vi "Turn Off All Outputs.vi"(8 "error in (no error)":errorcluster, 11 "Arduino in":refnum<class "Arduino.lvclass">) -> (0 "error out":errorcluster, 3 "Arduino out":refnum<class "Arduino.lvclass">)   [LabVIEW 2016, in "Arduino.lvclass"]
uses:
  Arduino.lvclass
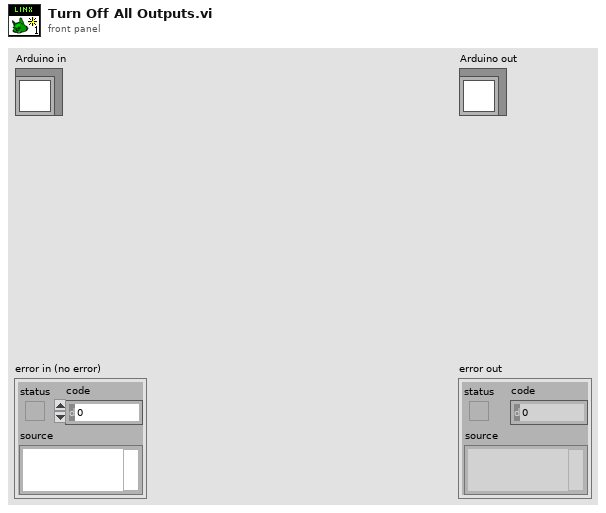
[diagram p1: front panel]
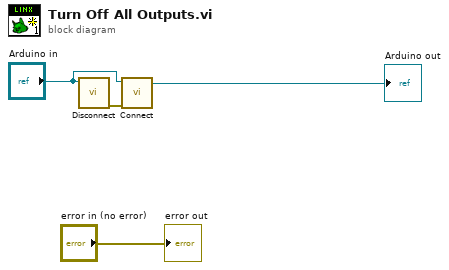
[diagram p0: block diagram]
diagram:
  n1 = call-dynamic "Disconnect.vi"("Arduino in"="Arduino in") -> ("error out"=w1:errorcluster)  [unwired: 9 in]
  n2 = call-dynamic "Connect.vi"("error in (no error)"=w1, "Arduino in"="Arduino in") -> ("Arduino out"=→"Arduino out":refnum<class "Arduino.lvclass">)  [unwired: 8 in, 1 out]
  "error out" <- "error in (no error)"
